vi "Disconnect.vi"(8 "error in (no error)":errorcluster, 11 "ClientBase in":refnum<class "ClientBase.lvclass">) -> (0 "error out":errorcluster, 3 "ClientBase out":refnum<class "ClientBase.lvclass">)   [LabVIEW 2020, in "ClientBaseLib.lvlib" / "ClientBase.lvclass"]
uses:
  ClientBase.lvclass
  ClientBase.lvclass/ClientBase.ctl
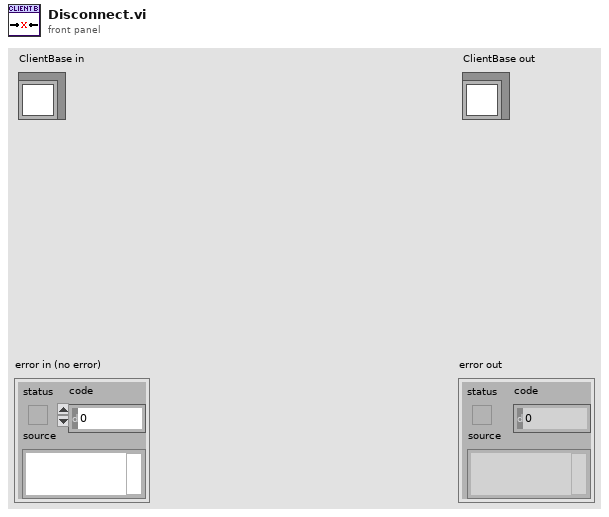
[diagram p1: front panel]
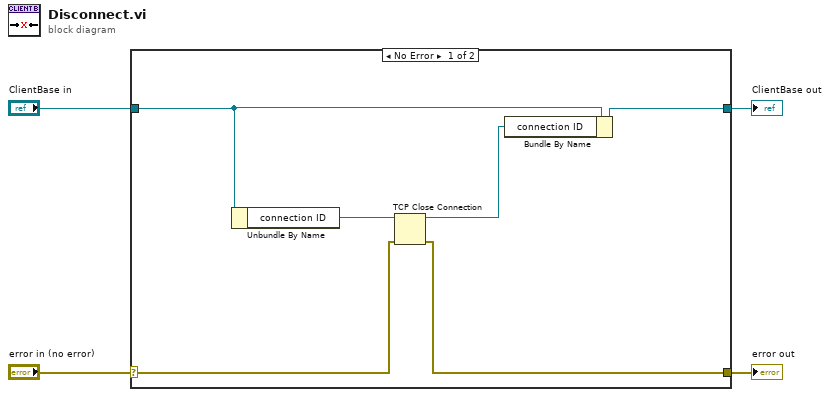
[diagram p0: block diagram]
diagram:
  n1 = case shown="No Error" "error in (no error)" {
    selector: "error in (no error)" -> [w6 w12]
    tunnel: [w5 w12] -> w3
    tunnel: [w8 w11] -> w1
    tunnel: "ClientBase in" -> [w10 w11]
    frame No Error {
      n2 = Unbundle By Name(w10) -> ("connection ID"=w9:refnum<k5>)
      n3 = TCP Close Connection(connection ID=w9, error in (no error)=w6) -> (connection ID out=w7:refnum<k5>, error out=w5:errorcluster)  [unwired: 1 in]
      n4 = Bundle By Name(cluster=w10, "connection ID"=w7) -> (w8:refnum<class "ClientBase.lvclass">)
    }
    frame Error {
    }
  }
  "error out" <- w3
  "ClientBase out" <- w1
